vi "Write path.vi"(8 "error in (no error)":errorcluster, 10 "path":path=path "c:/syslog.txt", 11 "Logger in":refnum<class "Logger.lvclass">) -> (0 "error out":errorcluster, 3 "Logger out":refnum<class "Logger.lvclass">)   [LabVIEW 2016, in "Logger.lvclass"]
uses:
  Logger.lvclass
  Logger.lvclass/Logger.ctl
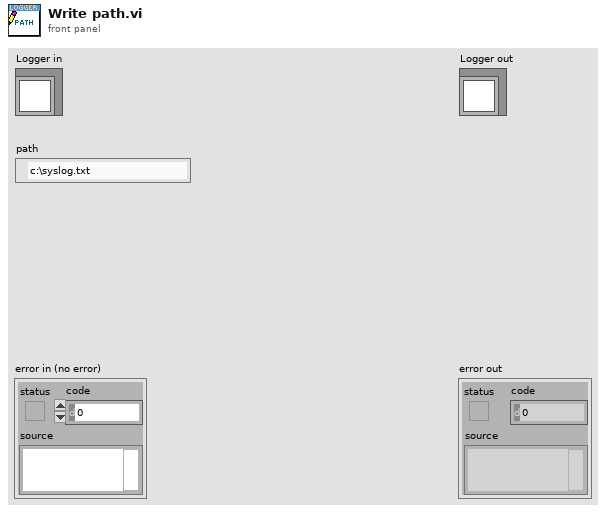
[diagram p1: front panel]
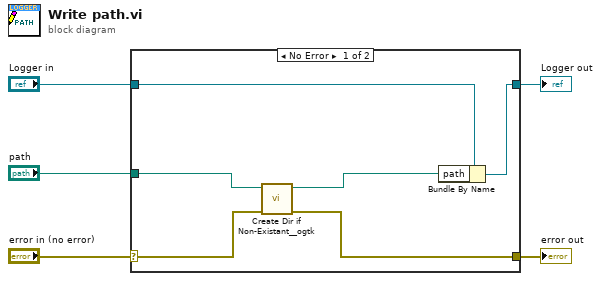
[diagram p0: block diagram]
diagram:
  n1 = case shown="No Error" "error in (no error)" {
    selector: "error in (no error)" -> [w9 w12]
    tunnel: [w6 w12] -> w4
    tunnel: [w10 w13] -> w2
    tunnel: "Logger in" -> [w11 w13]
    tunnel: "path" -> [w8 _]
    frame No Error {
      n2 = call <userlib>:"Create Dir if Non-Existant__ogtk.vi"("error in (no error)"=w9, "Directory Path"=w8) -> ("error out"=w6:errorcluster, "dup Directory Path"=w7:path)  [unwired: 7 in, 1 out]
      n3 = Bundle By Name(cluster=w11, "path"=w7) -> (w10:refnum<class "Logger.lvclass">)
    }
    frame Error {
    }
  }
  "error out" <- w4
  "Logger out" <- w2
